vi "Alerte_Temperature.vi"() -> ()   [LabVIEW 2018]
doc: "VI qui affiche des alertes (warnings) de température dans une station de météo. Ce VI est une partie du projet de Station Météo de Température, étudié durant la majorité des séances de TP."
panel:
  out "Message d'Avertissement":string
  out "Avertissement?":bool
  in  "Temp Min":dbl
  in  "Temp Max":dbl
  in  "Temp":dbl
  # "TP N°2"
  # "Mekni Marwen 2ème Année Génie Electrique"
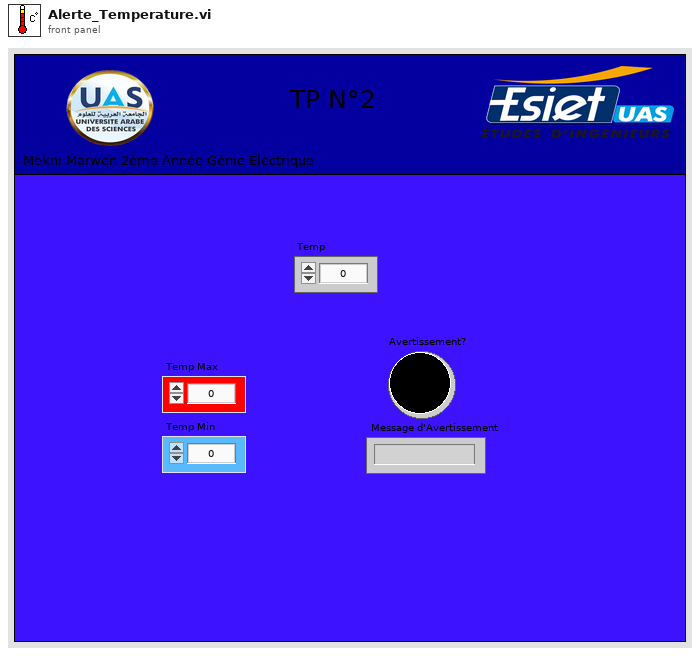
[diagram p1: front panel]
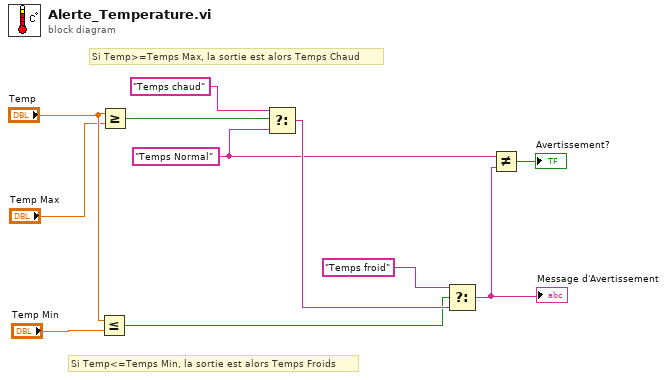
[diagram p0: block diagram]
diagram:
  w4 = "Temps Normal"
  # "Si Temp>=Temps Max, la sortie est alors Temps Chaud"
  # "Si Temp<=Temps Min, la sortie est alors Temps Froids"
  n1 = Less Or Equal?(x="Temp", y="Temp Min") -> (x <= y?=w5:bool)
  n2 = Greater Or Equal?(x="Temp", y="Temp Max") -> (x >= y?=w9:bool)
  n3 = Select(t="Temps chaud", s=w9, f=w4) -> (s? t:f=w7:string)
  n4 = Select(t="Temps froid", s=w5, f=w7) -> (s? t:f=w2:string)
  "Message d'Avertissement" <- w2
  n5 = Not Equal?(x=w4, y=w2) -> (x != y?=→"Avertissement?":bool)
